vi "Host_HoopingScan(NoXYCalculation).vi"() -> ()   [LabVIEW 2014]
uses:
  <vilib>/Native 3D Graph/xcontrol/3DPC_SurfacePlot.xctl
  <vilib>/FPGAPlugInAG/PCIe-7851R/niLvFpga_Open_PCIe-7851R.vi
  <vilib>/rvi/interface/common/dynamic/niFpgaDynamicAddResources.vi
  <vilib>/Utility/error.llb/Error Cluster From Error Code.vi
  <vilib>/rvi/errors/niLvFpgaAdjustHostInterfaceError.vi
  <vilib>/FPGAPlugInAG/Dynamic/niLvFpga_Close_Dynamic.vi
  <vilib>/rvi/interface/nirviOpenFPGA/nirviOpenFPGA.xnode
  FPGA Bitfiles/XZFPGAWithinHopp_FPGATarget_FPGAHoppingStep2_RD3GpH8S-LA.lvbitx
  <vilib>/rvi/interface/nirviMethod/nirviMethod.xnode
  <vilib>/rvi/interface/nirviReadWriteControl/nirviReadWriteControl.xnode
  <vilib>/rvi/interface/nirviCloseFPGA/nirviCloseFPGA.xnode
  <vilib>/FPGAPlugInAG/Dynamic/niLvFpga_WriteFifo_Dynamic.vi
  <vilib>/rvi/errors/niLvFpgaMergeErrorWithErrorCode.vi
  <vilib>/rvi/interface/Simulation/niFpgaSimulationCallBeginRW.vi
  <vilib>/FPGAPlugInAG/Dynamic/niLvFpga_ReadFifo_Dynamic.vi
  NiFpgaLv.dll
panel:
  out "x-y":u32
  out "XPresNum":u32
  out "YPresNum":i32
  out "ZHeight":refnum<class "Base Datatype.lvclass">[](xcontrol)
  out "ZPresPos":i16(graph)
  in  "stop":bool
  in  "Sleep us":i32
  in  "ZRelativeWithdraw":i16
  in  "ZOffsetIndex":i16
  in  "YOffsetIndex":i16
  in  "YStepIndex":i16
  in  "YNum":i16
  in  "XOffsetIndex":i16
  in  "XStepIndex":i16
  in  "XNum":i16
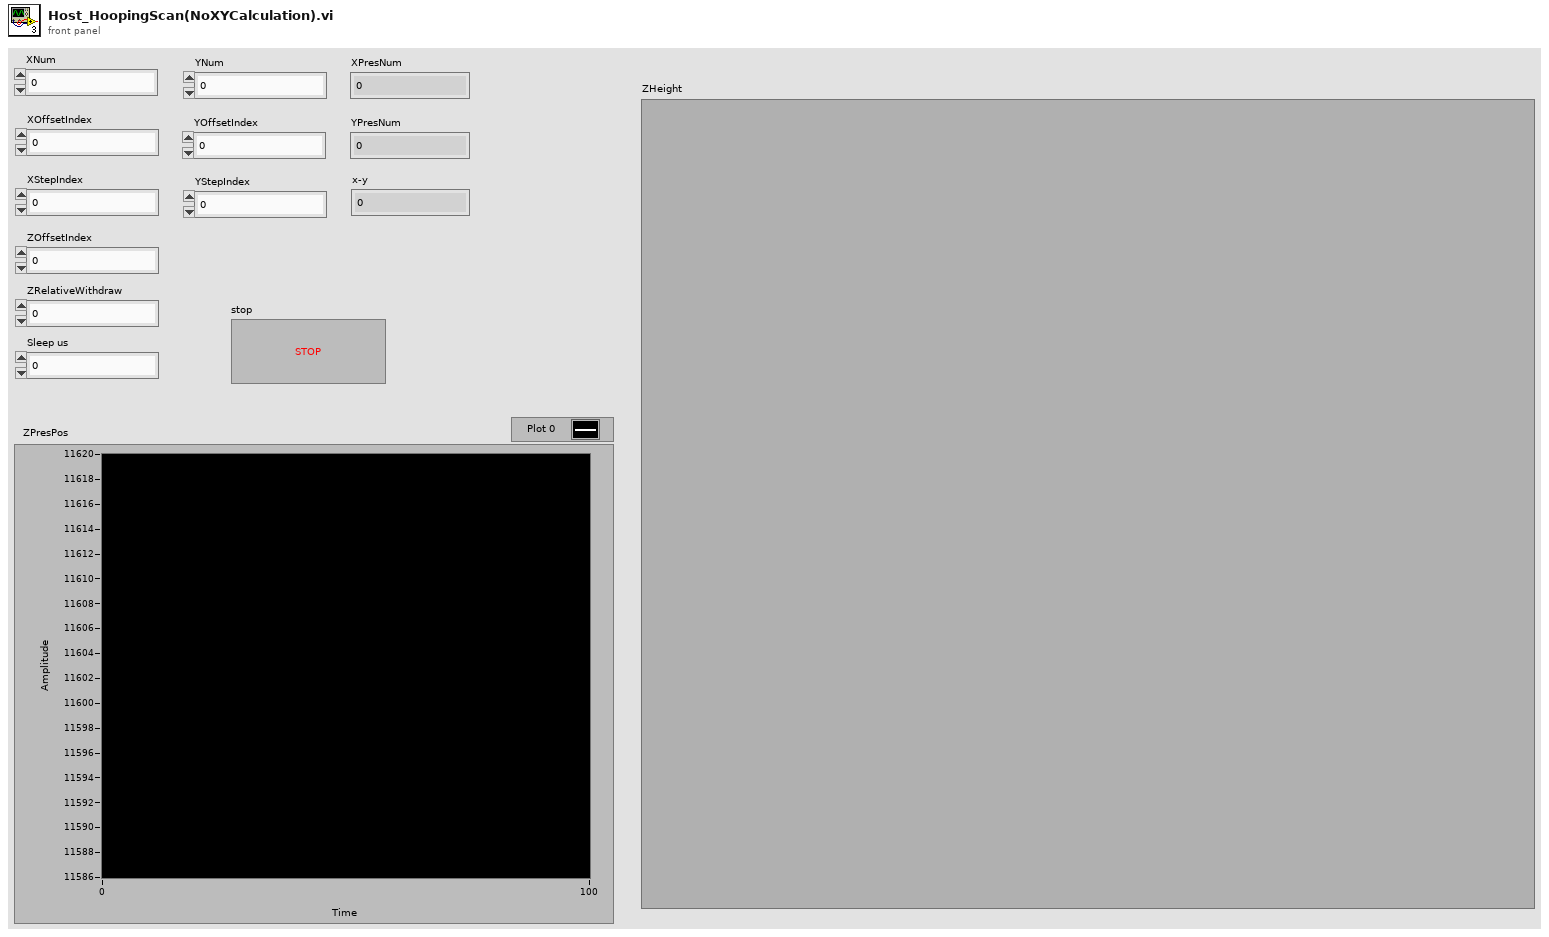
[diagram p1: front panel]
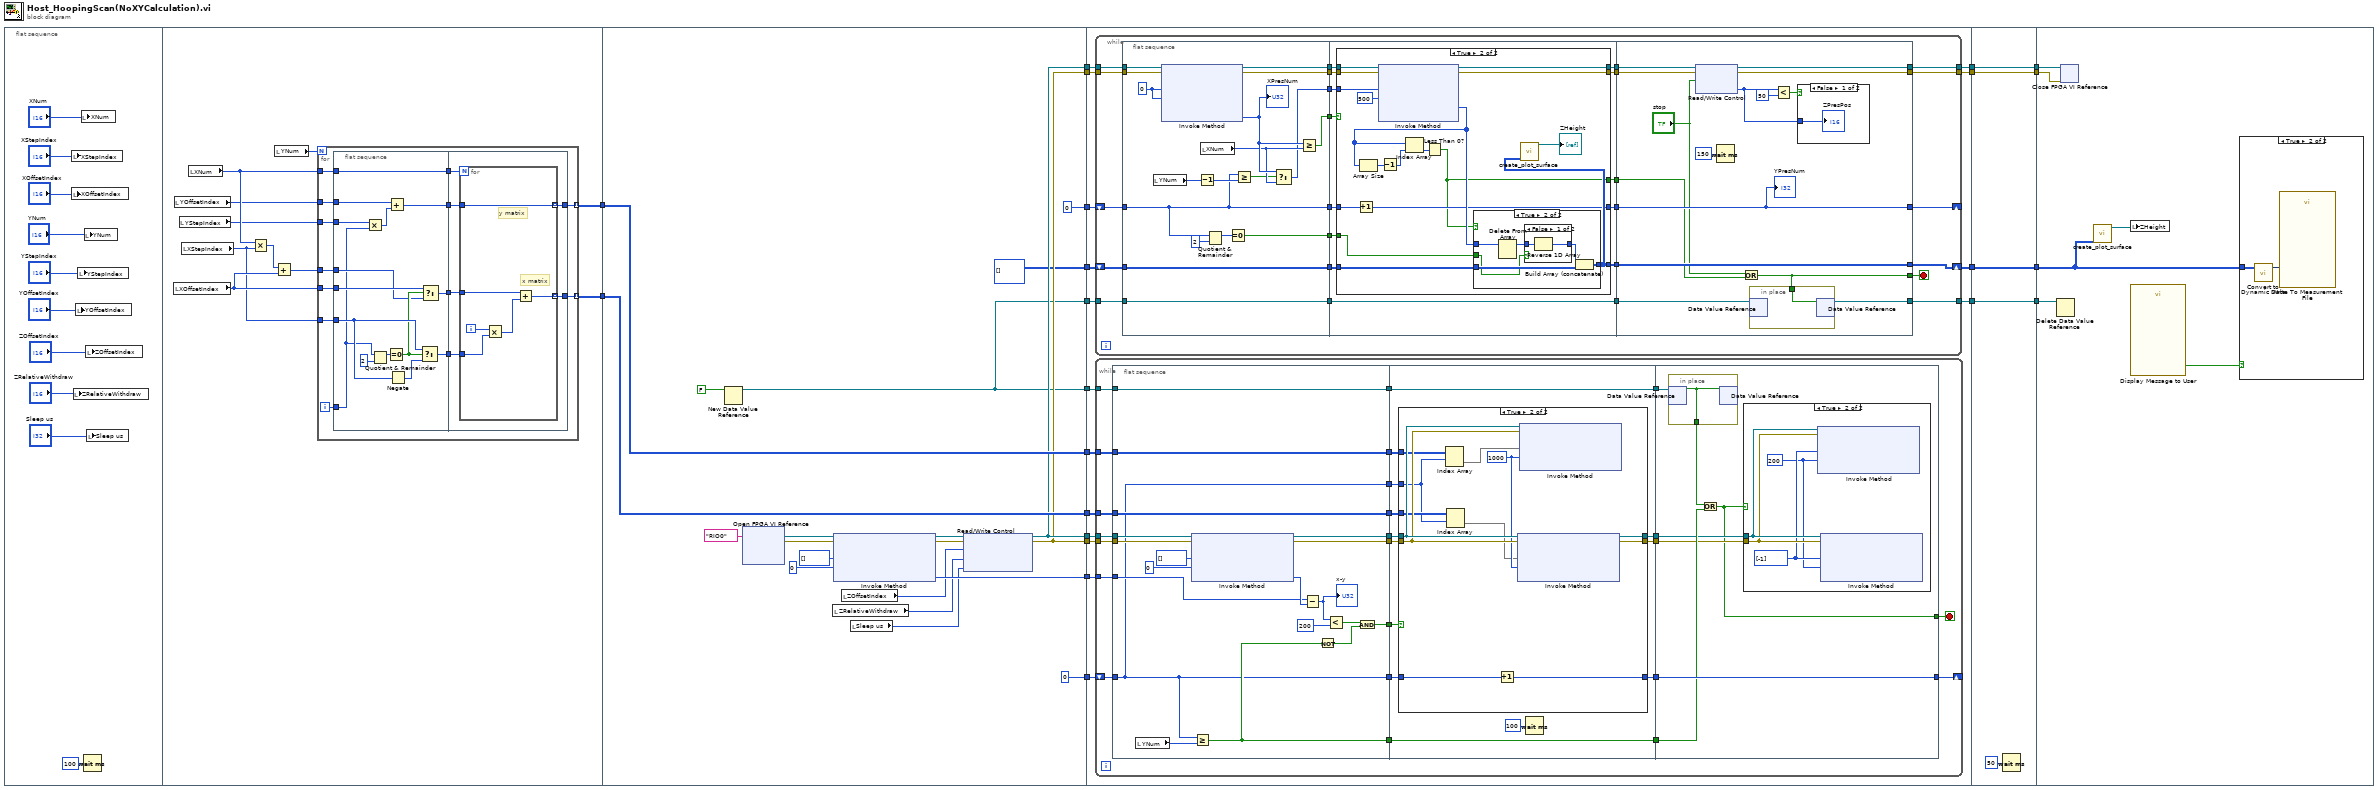
[diagram p0: block diagram]
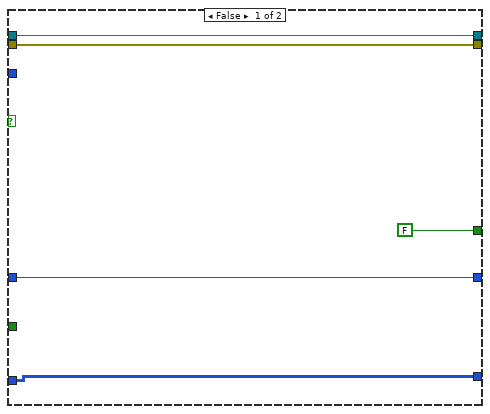
[diagram p4: hidden frame]
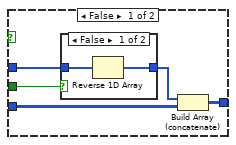
[diagram p5: hidden frame]
diagram:
  n1 = flat-sequence {
    tunnel: [w34] -> w18
    tunnel: [w33] -> w16
    tunnel: [w95] -> w22
    tunnel: [w87] -> w21
    tunnel: [w86] -> w20
    tunnel: [0 ("Timeout (ms)")] -> w19
    tunnel: w18 -> [w90]
    tunnel: [w90] -> w17
    tunnel: w16 -> [w89]
    tunnel: [w89] -> w15
    tunnel: [w83] -> w14
    tunnel: [w87] -> w13
    tunnel: [w86] -> w12
    tunnel: [0] -> w11
    tunnel: [i16[][] [] ("Data")] -> w10
    tunnel: [w83] -> w5
    tunnel: w22 -> [w116]
    tunnel: w21 -> [w118]
    tunnel: w20 -> [w117]
    tunnel: w19 -> [w115]
    tunnel: w17 -> [w114]
    tunnel: w15 -> [w113]
    tunnel: w14 -> [w112]
    tunnel: w13 -> [w111]
    tunnel: w12 -> [w110]
    tunnel: w11 -> [w109]
    tunnel: w10 -> [w108]
    tunnel: [w107] -> w9
    tunnel: [w106] -> w8
    tunnel: w5 -> [w105]
    tunnel: [w104] -> w4
    tunnel: [w103] -> w1
    tunnel: w9 -> [w317]
    tunnel: w8 -> [w316]
    tunnel: [w317] -> w7
    tunnel: [w316] -> w6
    tunnel: w4 -> [w314]
    tunnel: [w314] -> w3
    tunnel: [w313] -> w2
    tunnel: w1 -> [w313]
    tunnel: w7 -> [w323]
    tunnel: w6 -> [w322]
    tunnel: w3 -> [w321]
    tunnel: w2 -> [w319]
    frame #0 {
      n2 = local write "XStepIndex"("XStepIndex") -> ()
      n3 = local write "XOffsetIndex"("XOffsetIndex") -> ()
      n4 = local write "ZRelativeWithdraw"("ZRelativeWithdraw") -> ()
      n5 = local write "YOffsetIndex"("YOffsetIndex") -> ()
      n6 = local write "YStepIndex"("YStepIndex") -> ()
      n7 = local write "XNum"("XNum") -> ()
      n8 = Wait (ms)(milliseconds to wait=u32 100) -> ()  [unwired: 1 out]
      n9 = local write "YNum"("YNum") -> ()
      n10 = local write "ZOffsetIndex"("ZOffsetIndex") -> ()
      n11 = local write "Sleep us"("Sleep us") -> ()
    }
    frame #1 {
      n12 = local read "XOffsetIndex"() -> (w38:i16)
      n13 = local read "YOffsetIndex"() -> (w36:i16)
      n14 = local read "YStepIndex"() -> (w35:i16)
      n15 = local read "XStepIndex"() -> (w37:i16)
      n16 = local read "XNum"() -> (w41:i16)
      n17 = Multiply(x=w41, y=w37) -> (x*y=w40:i16)
      n18 = local read "YNum"() -> (w42:i16)
      n19 = Add(x=w40, y=w38) -> (x+y=w39:i16)
      n20 = for {
        N: w42 -> [_]
        tunnel: w41 -> [w55]
        tunnel: w39 -> [w53]
        tunnel: w38 -> [w52]
        tunnel: w37 -> [w50]
        tunnel: w36 -> [w47]
        tunnel: w35 -> [w46]
        tunnel: [w44] -> w33 mode=indexing
        tunnel: [w43] -> w34 mode=indexing
        i -> [w51]
        n21 = flat-sequence {
          tunnel: w55 -> [w70]
          tunnel: [w70] -> w54
          tunnel: w53 -> [w62]
          tunnel: w52 -> [w63]
          tunnel: w51 -> [w59]
          tunnel: w50 -> [w66]
          tunnel: [w65] -> w49
          tunnel: [w61] -> w48
          tunnel: w47 -> [w58]
          tunnel: w46 -> [w60]
          tunnel: [w56] -> w45
          tunnel: w54 -> [w76]
          tunnel: w49 -> [w75]
          tunnel: w48 -> [w74]
          tunnel: w45 -> [w73]
          tunnel: [w72] -> w44
          tunnel: [w71] -> w43
          frame #0 {
            n22 = Multiply(x=w60, y=w59) -> (x*y=w57:i32)
            n23 = Quotient & Remainder(x=w59, y=i16 2) -> (x-y*floor(x/y)=w68:i32)  [unwired: 1 out]
            n24 = Equal To 0?(x=w68) -> (x = 0?=w64:bool)
            n25 = Add(x=w58, y=w57) -> (x+y=w56:i32)
            n26 = Negate(x=w66) -> (-x=w67:i16)
            n27 = Select(t=w66, s=w64, f=w67) -> (s? t:f=w65:i16)
            n28 = Select(t=w63, s=w64, f=w62) -> (s? t:f=w61:i16)
          }
          frame #1 {
            n29 = for {
              N: w76 -> [_]
              tunnel: w75 -> [w81]
              tunnel: w74 -> [w80]
              tunnel: w73 -> [w77]
              tunnel: [w78] -> w71 mode=indexing
              tunnel: [w77] -> w72 mode=indexing
              i -> [w82]
              # "x matrix"
              # "y matrix"
              n30 = Multiply(x=w82, y=w81) -> (x*y=w79:i32)
              n31 = Add(x=w80, y=w79) -> (x+y=w78:i32)
            }
          }
        }
      }
    }
    frame #2 {
      n32 = New Data Value Reference(data value=FALSE) -> (data value reference=w83:refnum<data-value>)  [unwired: 1 in, 1 out]
      n33 = xnode ("Open FPGA VI Reference")("resource name"=tag "RIO0") -> ("FPGA VI Reference Out"=w101:refnum<k20>, "error out"=w100:errorcluster)  [unwired: 1 in]
      n34 = local read "ZRelativeWithdraw"() -> (w93:i16)
      n35 = xnode "Invoke Method"("FPGA VI Reference In"=w101, "error in"=w100, "Data"=i16[] [], "Timeout (ms)"=0) -> ("FPGA VI Reference Out"=w97:refnum<k20>, "error out"=w96:errorcluster, "Empty Elements Remaining"=w95:u32)
      n36 = local read "ZOffsetIndex"() -> (w94:i16)
      n37 = local read "Sleep us"() -> (w92:i32)
      n38 = xnode "Read/Write Control"("FPGA VI Reference In"=w97, "error in"=w96, "ZOffset"=w94, "RelativeWithdraw"=w93, "Sleep us"=w92) -> ("FPGA VI Reference Out"=w87:refnum<k20>, "error out"=w86:errorcluster)
    }
    frame #3 {
      n39 = while {
        tunnel: w111 -> [w225]
        tunnel: w110 -> [w224]
        shift-right: [w212] -> _
        shift-left: w109 -> [w223]
        shift-right: [w210] -> w103
        shift-left: w108 -> [w222]
        tunnel: [w214] -> w107
        tunnel: [w213] -> w106
        tunnel: w105 -> [w209]
        tunnel: [w205] -> w104
        stop <- w204 stop-if-true
        n40 = flat-sequence {
          tunnel: w225 -> [w243]
          tunnel: w224 -> [w242]
          tunnel: w223 -> [w230]
          tunnel: w222 -> [w240]
          tunnel: [w240] -> w221
          tunnel: [w239] -> w220
          tunnel: [w238] -> w219
          tunnel: [w230] -> w216
          tunnel: w209 -> [w237]
          tunnel: [w237] -> w208
          tunnel: [w234] -> w203
          tunnel: [w226] -> w202
          tunnel: [w233] -> w201
          tunnel: w221 -> [w251]
          tunnel: w220 -> [w256]
          tunnel: w219 -> [w255]
          tunnel: [w254] -> w218
          tunnel: [w253] -> w217
          tunnel: w216 -> [w252]
          tunnel: [w250] -> w215
          tunnel: [w249] -> w211
          tunnel: w208 -> [w248]
          tunnel: [w248] -> w207
          tunnel: [w247] -> w206
          tunnel: w203 -> [w246]
          tunnel: w202 -> [w245]
          tunnel: w201 -> [w244]
          tunnel: w218 -> [w308]
          tunnel: w217 -> [w307]
          tunnel: w215 -> [w310]
          tunnel: [w306] -> w214
          tunnel: [w305] -> w213
          tunnel: [w310] -> w212
          tunnel: w211 -> [w309]
          tunnel: [w309] -> w210
          tunnel: w207 -> [w302]
          tunnel: w206 -> [w303]
          tunnel: [w301] -> w205
          tunnel: [w296] -> w204
          frame #0 {
            w241 = 0
            n41 = local read "YNum"() -> (w232:i16)
            n42 = xnode "Invoke Method"("FPGA VI Reference In"=w243, "error in"=w242, "Number of Elements"=w241, "Timeout (ms)"=w241) -> ("FPGA VI Reference Out"=w239:refnum<k20>, "error out"=w238:errorcluster, "Elements Remaining"=w229:u32)  [unwired: 1 out]
            "XPresNum" <- w229
            n43 = Decrement(x=w232) -> (x-1=w231:i16)
            n44 = local read "XNum"() -> (w228:i16)
            n45 = Quotient & Remainder(x=w230, y=2) -> (x-y*floor(x/y)=w235:i32)  [unwired: 1 out]
            n46 = Equal To 0?(x=w235) -> (x = 0?=w234:bool)
            n47 = Greater Or Equal?(x=w230, y=w231) -> (x >= y?=w227:bool)
            n48 = Select(t=w229, s=w227, f=w228) -> (s? t:f=w226:u32)
            n49 = Greater Or Equal?(x=w229, y=w228) -> (x >= y?=w233:bool)
          }
          frame #1 {
            n50 = case shown="True" w244 {
              tunnel: w256 -> [w261 w278]
              tunnel: w255 -> [w260 w277]
              tunnel: [w261 w275] -> w254
              tunnel: [w260 w274] -> w253
              tunnel: w252 -> [w259 w265]
              tunnel: w251 -> [w258 w271]
              tunnel: [w259 w264] -> w250
              tunnel: [w258 w268] -> w249
              tunnel: [FALSE w263] -> w247
              tunnel: w246 -> [_ w267]
              tunnel: w245 -> [_ w266]
              frame False {
              }
              frame True {
                n51 = Increment(x=w265) -> (x+1=w264:i32)
                n52 = xnode "Invoke Method"("FPGA VI Reference In"=w278, "error in"=w277, "Number of Elements"=w266, "Timeout (ms)"=500) -> ("FPGA VI Reference Out"=w275:refnum<k20>, "error out"=w274:errorcluster, "Data"=w270:i16[])  [unwired: 1 out]
                n53 = Array Size(array=w270) -> (size(s)=w273:i32)
                n54 = Decrement(x=w273) -> (x-1=w262:i32)
                n55 = Index Array(array=w270, index=w262) -> (element=w272:i16)
                n56 = Less Than 0?(x=w272) -> (x < 0?=w263:bool)
                n57 = case shown="True" w263 {
                  tunnel: w271 -> [w283 w291]
                  tunnel: w270 -> [w281 w289]
                  tunnel: [w282 w290] -> w268
                  tunnel: w267 -> [w279 w287]
                  frame False {
                    n58 = case shown="False" w279 {
                      tunnel: w281 -> [w285 w286]
                      tunnel: [w284 w286] -> w280
                      frame False {
                        n59 = Reverse 1D Array(array=w285) -> (reversed array=w284:i16[])
                      }
                      frame True {
                      }
                    }
                    n60 = Build Array (concatenate)(w280, w283) -> (w282:i16[][])
                  }
                  frame True {
                    n61 = Delete From Array(array=w289) -> (array with subset deleted=w288:i16[])  [unwired: 2 in, 1 out]
                    n62 = case shown="False" w287 {
                      tunnel: w288 -> [w294 w295]
                      tunnel: [w293 w295] -> w292
                      frame False {
                        n63 = Reverse 1D Array(array=w294) -> (reversed array=w293:i16[])
                      }
                      frame True {
                      }
                    }
                    n64 = Build Array (concatenate)(w292, w291) -> (w290:i16[][])
                  }
                }
                n65 = call <vilib>:"create_plot_surface.vi"("z matrix"=w268) -> ("plots out"=→"ZHeight":refnum<class "Base Datatype.lvclass">[])  [unwired: 4 in, 6 out]
              }
            }
          }
          frame #2 {
            n66 = xnode "Read/Write Control"("FPGA VI Reference In"=w308, "error in"=w307, "stop"="stop") -> ("FPGA VI Reference Out"=w306:refnum<k20>, "error out"=w305:errorcluster, "ZPresPos"=w297:i16)
            n67 = Wait (ms)(milliseconds to wait=u32 150) -> ()  [unwired: 1 out]
            n68 = Or(x="stop", y=w303) -> (x .or. y?=w296:bool)
            n69 = in-place {
              in-place-border: w296 -> [w312]
              n70 = in-place-dvr #1(w302) -> ()  [unwired: 2 out]
              n71 = in-place-dvr #1(w312) -> (w301:refnum<data-value>)  [unwired: 1 out]
            }
            n72 = Less?(x=w297, y=i16 50) -> (x < y?=w299:bool)
            n73 = case shown="False" w299 {
              tunnel: w297 -> [w311 _]
              frame False {
                "ZPresPos" <- w311
              }
              frame True {
              }
            }
            "YPresNum" <- w310
          }
        }
      }
      n74 = while {
        tunnel: w118 -> [w141]
        tunnel: w117 -> [w140]
        tunnel: w116 -> [w139]
        shift-right: [w125] -> _
        shift-left: w115 -> [w138]
        tunnel: w114 -> [w130]
        tunnel: w113 -> [w129]
        tunnel: w112 -> [w122]
        stop <- w119 stop-if-true
        n75 = flat-sequence {
          tunnel: w141 -> [w160]
          tunnel: w140 -> [w159]
          tunnel: w139 -> [w155]
          tunnel: w138 -> [w143]
          tunnel: [w143] -> w137
          tunnel: [w149] -> w136
          tunnel: [w148] -> w134
          tunnel: [w147] -> w133
          tunnel: [w146] -> w132
          tunnel: [w145] -> w131
          tunnel: w130 -> [w145]
          tunnel: w129 -> [w144]
          tunnel: [w144] -> w128
          tunnel: [w143] -> w127
          tunnel: w122 -> [w142]
          tunnel: [w142] -> w121
          tunnel: w137 -> [w173]
          tunnel: w136 -> [w172]
          tunnel: [w172] -> w135
          tunnel: w134 -> [w170]
          tunnel: w133 -> [w169]
          tunnel: w132 -> [w168]
          tunnel: w131 -> [w167]
          tunnel: w128 -> [w166]
          tunnel: w127 -> [w165]
          tunnel: [w164] -> w126
          tunnel: [w163] -> w124
          tunnel: [w162] -> w123
          tunnel: w121 -> [w161]
          tunnel: [w161] -> w120
          tunnel: w135 -> [w192]
          tunnel: w126 -> [w195]
          tunnel: [w195] -> w125
          tunnel: w124 -> [w191]
          tunnel: w123 -> [w190]
          tunnel: w120 -> [w194]
          tunnel: [w189] -> w119
          frame #0 {
            n76 = local read "YNum"() -> (w151:i16)
            n77 = xnode "Invoke Method"("FPGA VI Reference In"=w160, "error in"=w159, "Data"=i16[] [], "Timeout (ms)"=0) -> ("FPGA VI Reference Out"=w147:refnum<k20>, "error out"=w146:errorcluster, "Empty Elements Remaining"=w156:u32)
            n78 = Greater Or Equal?(x=w143, y=w151) -> (x >= y?=w149:bool)
            n79 = Subtract(x=w155, y=w156) -> (x-y=w154:u32)
            "x-y" <- w154
            n80 = Not(x=w149) -> (.not. x?=w150:bool)
            n81 = Less?(x=w154, y=u32 200) -> (x < y?=w152:bool)
            n82 = And(x=w152, y=w150) -> (x .and. y?=w148:bool)
          }
          frame #1 {
            n83 = case shown="True" w170 {
              tunnel: w173 -> [w176 w180]
              tunnel: w169 -> [w175 w188]
              tunnel: w168 -> [w174 w187]
              tunnel: w167 -> [_ w184]
              tunnel: w166 -> [_ w185]
              tunnel: w165 -> [_ w183]
              tunnel: [w176 w179] -> w164
              tunnel: [w175 w178] -> w163
              tunnel: [w174 w177] -> w162
              frame False {
              }
              frame True {
                w186 = 1000 ("Timeout (ms)")
                n84 = Index Array(array=w185, index (row)=w183) -> (element=w182:i32[])  [unwired: 1 in]
                n85 = Index Array(array=w184, index (row)=w183) -> (element=w181:i32[])  [unwired: 1 in]
                n86 = Increment(x=w180) -> (x+1=w179:i32)
                n87 = xnode "Invoke Method"("FPGA VI Reference In"=w188, "error in"=w187, "Data"=w181, "Timeout (ms)"=w186) -> ("FPGA VI Reference Out"=w178:refnum<k20>, "error out"=w177:errorcluster)  [unwired: 1 out]
                n88 = xnode "Invoke Method"("FPGA VI Reference In"=w188, "error in"=w187, "Data"=w182, "Timeout (ms)"=w186) -> ()  [unwired: 3 out]
              }
            }
            n89 = Wait (ms)(milliseconds to wait=u32 100) -> ()  [unwired: 1 out]
          }
          frame #2 {
            n90 = in-place {
              in-place-border: [w200] -> w193
              n91 = in-place-dvr #2(w194) -> (w200:bool)  [unwired: 1 out]
              n92 = in-place-dvr #2(w200) -> ()  [unwired: 2 out]
            }
            n93 = Or(x=w193, y=w192) -> (x .or. y?=w189:bool)
            n94 = case shown="True" w189 {
              tunnel: w191 -> [_ w199]
              tunnel: w190 -> [_ w198]
              frame False {
              }
              frame True {
                w196 = 200 ("Timeout (ms)")
                w197 = i16[] [-1] ("Data")
                n95 = xnode "Invoke Method"("FPGA VI Reference In"=w199, "error in"=w198, "Data"=w197, "Timeout (ms)"=w196) -> ()  [unwired: 3 out]
                n96 = xnode "Invoke Method"("FPGA VI Reference In"=w199, "error in"=w198, "Data"=w197, "Timeout (ms)"=w196) -> ()  [unwired: 3 out]
              }
            }
          }
        }
      }
    }
    frame #4 {
      n97 = Wait (ms)(milliseconds to wait=u32 50) -> ()  [unwired: 1 out]
    }
    frame #5 {
      n98 = Delete Data Value Reference(data value reference=w321) -> ()  [unwired: 1 in, 2 out]
      n99 = xnode "Close FPGA VI Reference"("FPGA VI Reference In"=w323, "error in"=w322) -> ()  [unwired: 1 out]
      n100 = call <vilib>:"create_plot_surface.vi"("z matrix"=w319) -> ("plots out"=w318:refnum<class "Base Datatype.lvclass">[])  [unwired: 4 in, 6 out]
      n101 = local write "ZHeight"(w318) -> ()
      n102 = call "Display Message to User"() -> ("OK"=w320:bool)  [unwired: 10 in, 1 out]
      n103 = case shown="True" w320 {
        tunnel: w319 -> [_ w325]
        frame False {
        }
        frame True {
          n104 = call "Convert to Dynamic Data"("2D Array"=w325) -> ("Dynamic Data Type"=w324:dynamicdata)  [unwired: 3 in]
          n105 = call "Write To Measurement File"("Signals"=w324) -> ()  [unwired: 16 in, 3 out]
        }
      }
    }
  }
